vi "ALTS-2015 Write Users v1.1.vi"(8 "error in (no error)":errorcluster, 9 "User Group":T1, 10 "Password":string, 11 "User Name":string="Administrator") -> (0 "error out":errorcluster)   [LabVIEW 2013]
doc: "This VI is particularly used to write the information of a particular user."
uses:
  Controls/ALTS-2015 User Group Enum2.ctl
  Controls/ALTS-2015 User Info.ctl
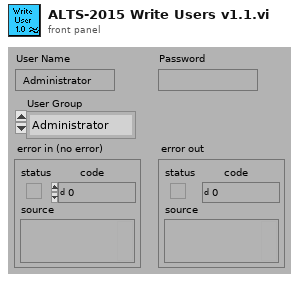
[diagram p1: front panel]
types:
  T1 = typedef "ALTS-2015 User Group Enum2.ctl" = enum16{"Administrator", "Super User", "Operator"}
  T2 = typedef "ALTS-2015 User Info.ctl" = cluster{"User Name":string, "Password":string, "User Right":T1}
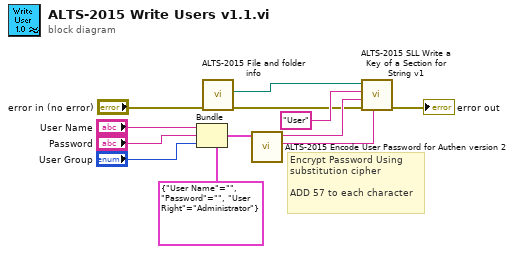
[diagram p0: block diagram]
diagram:
  # "Encrypt Password Using\nsubstitution cipher\n\nADD 57 to each character"
  n1 = Bundle(cluster=T2 {"User Name"="", "Password"="", "User Right"=enum."Administrator"} ("User Info"), "User Name"="User Name", "Password"="Password", "User Right"="User Group") -> (w5:T2)
  n2 = call "ALTS-2015 File and folder info.vi"("error in (no error)"="error in (no error)") -> ("error out"=w3:errorcluster, "INI file path"=w1:path)  [unwired: 5 in, 4 out]
  n3 = call "ALTS-2015 Encode User Password for Authen version 2.vi"("User Info"=w5) -> ("User Value (encoded)"=w4:string, "User Name"=w10:string)  [unwired: 9 in]
  n4 = call "ALTS-2015 SLL Write a Key of a Section for String v1.vi"("Key Value"=w4, "error in (no error)"=w3, "Key Name"=w10, "Section"="User", "Application INI file path"=w1) -> ("error out"=→"error out":errorcluster)  [unwired: 6 in]
